vi "Main.vi"() -> ()   [LabVIEW 2021]
uses:
  Data Source Type.ctl
  Scale/Scale.lvclass
  C:/PPLs/Decorator-Pattern/decorator-main/Presentation/Decorator/Decorator.lvclass
  LP Filter/LP Filter.lvclass
  File Reader/File Reader.lvclass
  C:/PPLs/Decorator-Pattern/decorator-main/Presentation/Component/Component.lvclass
  Normalize/Normalize.lvclass
  Function Generator/Function Generator.lvclass
  Component/Component.lvclass
  Decorator/Decorator.lvclass
panel:
  in  "Data Source Type":T1
  out "Data":dbl[][](graph)
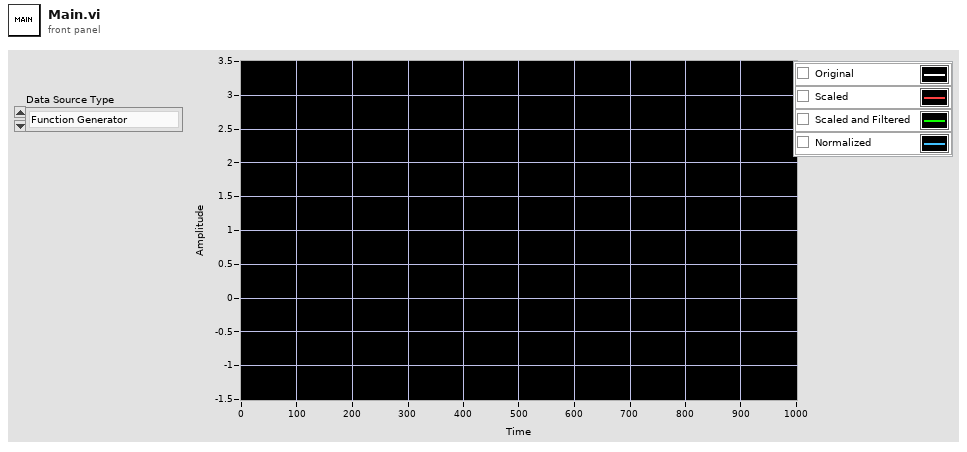
[diagram p1: front panel]
types:
  T1 = typedef "Data Source Type.ctl" = enum16{"Function Generator", "File"}
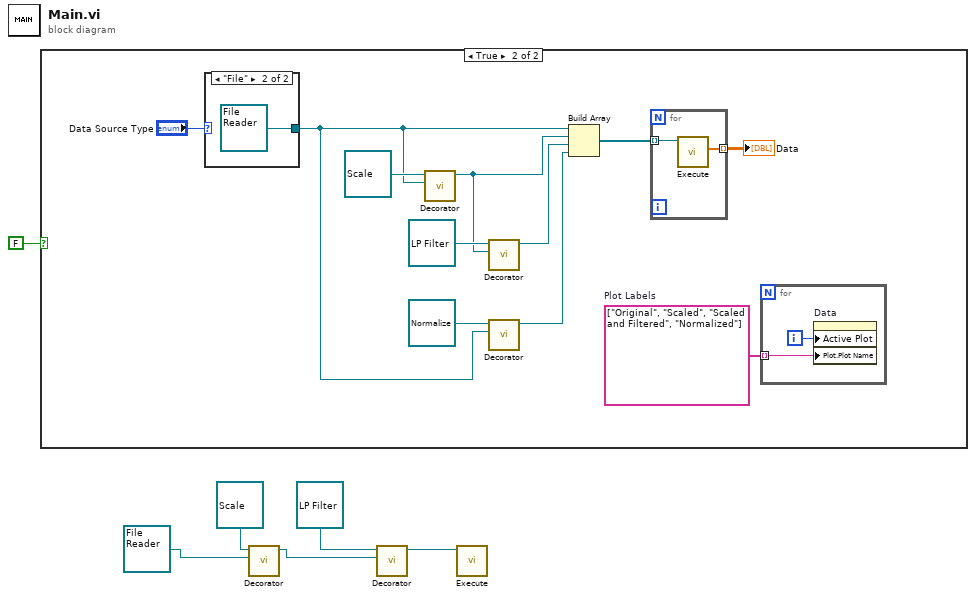
[diagram p0: block diagram]
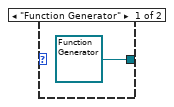
[diagram p3: hidden frame]
diagram:
  n1 = case shown="True" FALSE {
    frame False {
    }
    frame True {
      w14 = string[] ["Original", "Scaled", "Scaled and Filtered", "Normalized"]  # Plot Labels
      n2 = case shown="\"File\"" "Data Source Type" {
        tunnel: [refnum<class "Function Generator.lvclass"> refnum ("Function Generator.lvclass") refnum<class "File Reader.lvclass"> refnum ("File Reader")] -> w8
        frame "Function Generator" {
        }
        frame "File" {
        }
      }
      n3 = call "Decorator.vi"("Component"=w8, "Decorator in"=refnum<class "Scale.lvclass"> refnum ("Scale.lvclass")) -> ("Decorator out"=w12:refnum<class "Component.lvclass">)  [unwired: 9 in]
      n4 = call "Decorator.vi"("Component"=w12, "Decorator in"=refnum<class "LP Filter.lvclass"> refnum ("LP Filter.lvclass")) -> ("Decorator out"=w11:refnum<class "Component.lvclass">)  [unwired: 9 in]
      n5 = call "Decorator.vi"("Component"=w8, "Decorator in"=refnum<class "Normalize.lvclass"> refnum ("Normalize.lvclass")) -> ("Decorator out"=w10:refnum<class "Component.lvclass">)  [unwired: 9 in]
      n6 = Build Array(w8, w12, w11, w10) -> (w16:refnum<class "Component.lvclass">[])
      n7 = for {
        tunnel: w16 -> [w23] mode=indexing
        tunnel: [w22] -> w15 mode=indexing
        n8 = call-dynamic "Execute.vi"("Data Source in"=w23) -> ("Data"=w22:dbl[])  [unwired: 8 in, 2 out]
      }
      "Data" <- w15
      n9 = for {
        tunnel: w14 -> [w21] mode=indexing
        i -> [w20]
        n10 = property on="Data" class="WFGraph (strict)"("Active Plot"=w20, "Plot.Plot Name"=w21) -> ()  [unwired: 2 in, 2 out]
      }
    }
  }
  n11 = call "Decorator.vi"("Component"=refnum<class "File Reader.lvclass"> refnum ("File Reader"), "Decorator in"=refnum<class "Scale.lvclass"> refnum ("Scale.lvclass")) -> ("Decorator out"=w6:refnum<class "Component.lvclass">)  [unwired: 9 in]
  n12 = call "Decorator.vi"("Component"=w6, "Decorator in"=refnum<class "LP Filter.lvclass"> refnum ("LP Filter.lvclass")) -> ("Decorator out"=w2:refnum<class "Component.lvclass">)  [unwired: 9 in]
  n13 = call-dynamic "Execute.vi"("Data Source in"=w2) -> ()  [unwired: 8 in, 3 out]
